vi "ClassName.vi"(6 "error in":errorcluster, 9 "CaseStructure in":refnum<class "CaseStructure.lvclass">) -> (0 "error out":errorcluster, 3 "CaseStructure out":refnum<class "CaseStructure.lvclass">, 4 "class name":string)   [LabVIEW 2014, in "CaseStructure.lvclass"]
uses:
  CaseStructure.lvclass
  <vilib>/Utility/VariantDataType/VariantType.lvlib
panel:
  in  "module name":string="lvStruct"
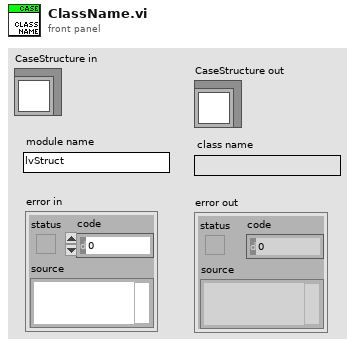
[diagram p1: front panel]
types:
  T1 = typedef "VariantType.lvlib/Type.ctl" = enum8{"Invalid Type", "Void", "I8", "I16", "I32", "I64", "U8", "U16", "U32", "U64", "Single Float", "Double Float", "Extended Float", "Single Complex", "Double Complex", "Extended Complex", "Enum U8", "Enum U16", "Enum U32", "Enum U64", "Single Float With Unit", "Double Float With Unit", "Extended Float With Unit", "Single Complex with Unit", "Double Complex with Unit", "Extended Complex with Unit", "Boolean", "String", "Path", "Picture", "Tag", "Array", "Cluster", "Variant", "LV Variant", "Waveform", "Timestamp", "Digital Waveform", "Digital Data", "ExpressData", "Refnum", "External Data", "VI", "Poly VI", "LabVIEW Class Instance", "Fixed Point"}
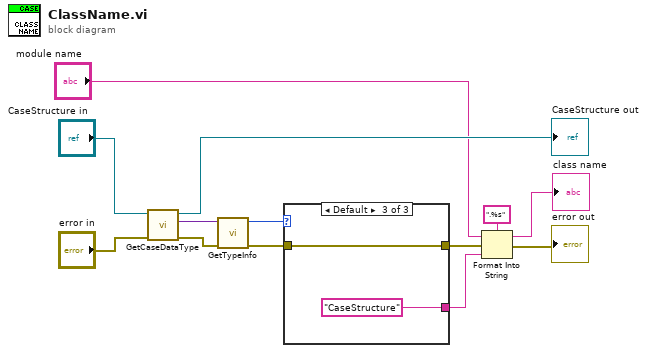
[diagram p0: block diagram]
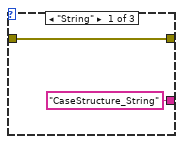
[diagram p2: hidden frame]
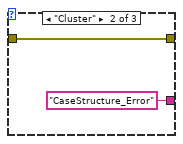
[diagram p3: hidden frame]
diagram:
  n1 = call "GetCaseDataType.vi"("error in"="error in", "CaseStructure in"="CaseStructure in") -> ("error out"=w11:errorcluster, "Data Type"=w12:variant, "CaseStructure out"=→"CaseStructure out":refnum<class "CaseStructure.lvclass">)  [unwired: 5 in]
  n2 = call <vilib>:"GetTypeInfo.vi"("error in (no error)"=w11, "Variant"=w12) -> ("error out"=w9:errorcluster, "Type Enum"=w10:T1)  [unwired: 5 in, 3 out]
  n3 = case shown="Default" w10 {
    tunnel: w9 -> [w15 w17 w19]
    tunnel: [w15 w17 w19] -> w5
    tunnel: ["CaseStructure_String" "CaseStructure_Error" "CaseStructure"] -> w3
    frame "String" {
    }
    frame "Cluster" {
    }
    frame Default {
    }
  }
  n4 = Format Into String(format string=".%s", initial string="module name", error in=w5, w3) -> (resulting string=→"class name":string, error out=→"error out":errorcluster)
